vi "create Series.vi"(8 "error in (no error)":errorcluster, 11 "Series":T1={"ChartType"=18, "Name"="", "Palette"=enum."Bright", "BorderDashStyle"=enum."Solid", "YAxisType"=enum."Secondary", "XAxisType"=enum."Primary", "BorderColor"=0, "Thickness"=0.0, "Color"=11711154, "Alpha"=76, "Marker"={"MarkerStyle"=enum."Triangle", "Size"=12, "Color"=0, "Step"=12}} {"Alpha" scale=0.0..255.0; "ChartType" items=["Point", "FastPoint", "Bubble", "Line", "Spline", "StepLine", "FastLine", "Bar", "StackedBar", "StackedBar100", "Column", "StackedColumn", "StackedColumn100", "Area", "SplineArea", "StackedArea", "StackedArea100", "Pie", "Doughnut", "Stock", "Candlestick", "Range", "SplineRange", "RangeBar", "RangeColumn", "Radar", "Polar", "ErrorBar", "BoxPlot", "Renko", "ThreeLineBreak", "Kagi", "PointAndFigure", "Funnel", "Pyramid"]}) -> (0 "error out":errorcluster, 3 ".net MSChart Series":refnum<k24>)   [LabVIEW 2015, in "Graph Extensions MSChart.lvlib"]
uses:
  Graph Extensions MSChart.lvlib
  System.Windows.Forms.DataVisualization
  Controls/Series.ctl
  Controls/Marker.ctl
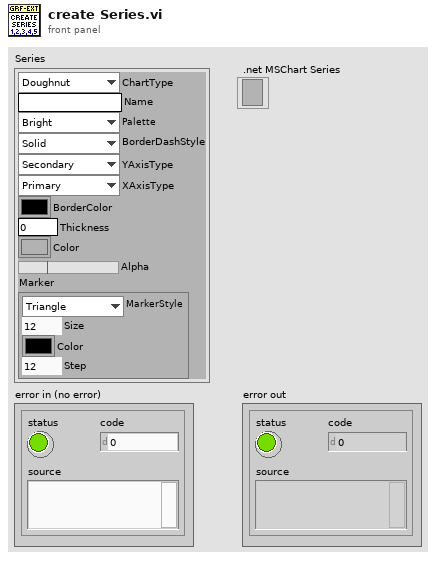
[diagram p1: front panel]
types:
  T1 = typedef "Graph Extensions MSChart.lvlib/Series.ctl" = cluster{"ChartType":i32, "Name":string, "Palette":enum16{"None", "Bright", "Grayscale", "Excel", "Light", "Pastel", "EarthTones", "SemiTransparent", "Berry", "Chocolate", "Fire", "SeaGreen", "BrightPastel"}, "BorderDashStyle":enum16{"NotSet", "Dash", "DashDot", "DashDotDot", "Dot", "Solid"}, "YAxisType":enum16{"Primary", "Secondary"}, "XAxisType":enum16{"Primary", "Secondary"}, "BorderColor":u32, "Thickness":dbl, "Color":u32, "Alpha":u8, "Marker":T2}
  T2 = typedef "Graph Extensions MSChart.lvlib/Marker.ctl" = cluster{"MarkerStyle":enum16{"None", "Square", "Circle", "Diamond", "Triangle", "Cross", "Star4", "Star5", "Star6", "Star10"}, "Size":i32, "Color":u32, "Step":i32}
  T3 = enum16{"None", "Bright", "Grayscale", "Excel", "Light", "Pastel", "EarthTones", "SemiTransparent", "Berry", "Chocolate", "Fire", "SeaGreen", "BrightPastel"}
  T4 = enum16{"NotSet", "Dash", "DashDot", "DashDotDot", "Dot", "Solid"}
  T5 = enum16{"None", "Square", "Circle", "Diamond", "Triangle", "Cross", "Star4", "Star5", "Star6", "Star10"}
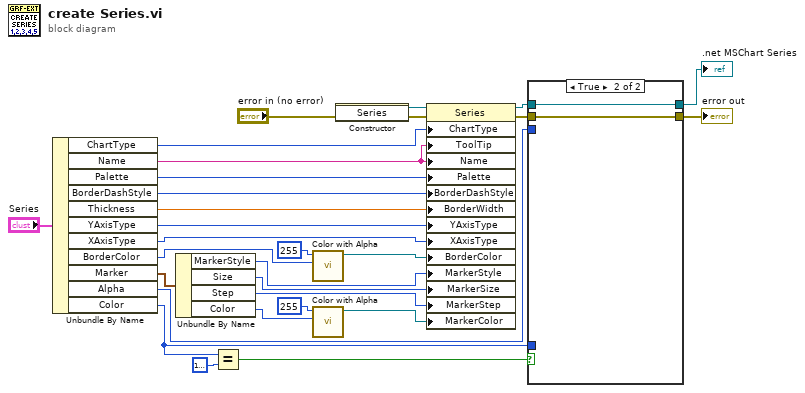
[diagram p0: block diagram]
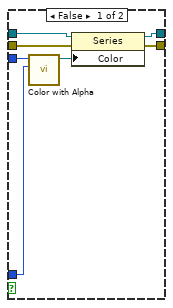
[diagram p2: hidden frame]
diagram:
  n1 = Unbundle By Name("Series") -> ("ChartType"=w9:i32, "Name"=w13:string, "Palette"=w24:T3, "BorderDashStyle"=w23:T4, "Thickness"=w10:dbl, "YAxisType"=w19:enum16{"Primary", "Secondary"}, "XAxisType"=w18:enum16{"Primary", "Secondary"}, "BorderColor"=w22:u32, "Marker"=w20:T2, "Alpha"=w8:u8, "Color"=w2:u32)
  n2 = Unbundle By Name(w20) -> ("MarkerStyle"=w17:T5, "Size"=w12:i32, "Step"=w11:i32, "Color"=w15:u32)
  n3 = Equal?(x=w2, y=u32 16777216) -> (x = y?=w1:bool)
  n4 = call "Color with Alpha.vi"("Color"=w22, "alpha"=255) -> (".NET color Refnum out"=w29:refnum<k24>)  [unwired: 9 in]
  n5 = call "Color with Alpha.vi"("Color"=w15, "alpha"=255) -> (".NET color Refnum out"=w14:refnum<k24>)  [unwired: 9 in]
  n6 = constructor class="Series"(error in="error in (no error)") -> (reference out=w27:refnum<k24>, error out=w28:errorcluster)  [unwired: 2 in, 1 out]
  n7 = property class="Series"(reference=w27, error in=w28, "ChartType"=w9, "ToolTip"=w13, "Name"=w13, "Palette"=w24, "BorderDashStyle"=w23, "BorderWidth"=w10, "YAxisType"=w19, "XAxisType"=w18, "BorderColor"=w29, "MarkerStyle"=w17, "MarkerSize"=w12, "MarkerStep"=w11, "MarkerColor"=w14) -> (reference out=w7:refnum<k24>, error out=w5:errorcluster)
  n8 = case shown="True" w1 {
    tunnel: w8 -> [w36 _]
    tunnel: w2 -> [w35 _]
    tunnel: w7 -> [w33 w38]
    tunnel: [w32 w38] -> w6
    tunnel: w5 -> [w31 w37]
    tunnel: [w30 w37] -> w4
    frame False {
      n9 = call "Color with Alpha.vi"("Color"=w35, "alpha"=w36) -> (".NET color Refnum out"=w34:refnum<k24>)  [unwired: 9 in]
      n10 = property class="Series"(reference=w33, error in=w31, "Color"=w34) -> (reference out=w32:refnum<k24>, error out=w30:errorcluster)
    }
    frame True {
    }
  }
  "error out" <- w4
  ".net MSChart Series" <- w6
